vi "Keithley 6517A Measure Query.vi"(3 "error in":T1, 4 "function (Vdc:0)":u16(ring)=1 items=["dc voltage", "dc current", "resistance", "charge"], 5 "GPIB Address":string="27") -> (0 "error out":T1, 1 "Reading Result":string)   [LabVIEW 2013]
doc: "You must turn ZERO CHECK off before you run this VI, otherwise, you will get the standard IEEE488.2 response for overflow (9.9E37). The VI returns the result of a SCPI Signal Oriented MEASURE? command. This is equivalent to a one shot reading.\n\nThis is a basic VI for getting readings back and is not necessarily the best method but rather a quick way to getting measurements."
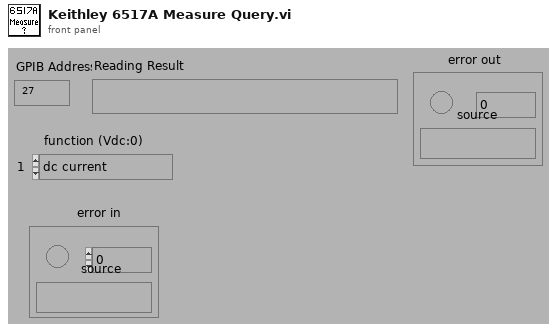
[diagram p1: front panel]
types:
  T1 = cluster{"error":bool, "code":i32, "source":string}
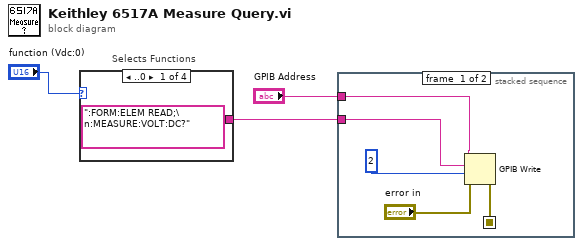
[diagram p0: block diagram]
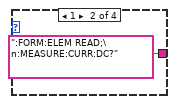
[diagram p2: hidden frame]
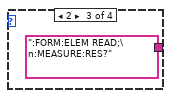
[diagram p3: hidden frame]
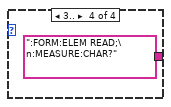
[diagram p4: hidden frame]
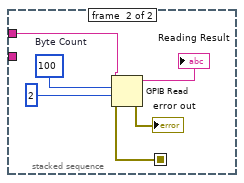
[diagram p5: hidden frame]
diagram:
  n1 = case "Selects Functions" shown="..0" "function (Vdc:0)" {
    tunnel: [":FORM:ELEM READ;\n:MEASURE:VOLT:DC?" ":FORM:ELEM READ;\n:MEASURE:CURR:DC?" ":FORM:ELEM READ;\n:MEASURE:RES?" ":FORM:ELEM READ;\n:MEASURE:CHAR?"] -> w1
    frame ..0 {
    }
    frame 1 {
    }
    frame 2 {
    }
    frame 3.. {
    }
  }
  n2 = stacked-sequence {
    seq-local: [w8 _] -> [_ w14]
    tunnel: "GPIB Address" -> [w9 w16]
    tunnel: w1 -> [w10 _]
    frame #0 {
      n3 = GPIB Write(0:w9, 1:w10, 2:2, 3:"error in") -> (6:w8:errorcluster)  [unwired: 1 in, 1 out]
    }
    frame #1 {
      w17 = 100  # Byte Count
      n4 = GPIB Read(0:w16, 1:w17, 2:2, 3:w14) -> (5:→"Reading Result":string, 7:→"error out":errorcluster)  [unwired: 1 in, 1 out]
    }
  }
